vi "_053.vi"() -> ()   [LabVIEW 2024]
uses:
  <vilib>/Math Plots/3D Math Plots/3D Bar/3D Bar XCtrl/3D Bar.xctl
  <vilib>/Math Plots/3D Math Plots/3D Bar/3D Bar Datatype/Public/Plot Helper (Matrix).vi
  <vilib>/Math Plots/3D Math Plots/3D Bar/3D Bar Datatype/3D Bar Datatype.lvclass
panel:
  out "3D Bar":refnum<class "3D Plot Datatype.lvclass">[](xcontrol)
  # "Data plot on 3D Bar Graph :"
  # "( Sin & Cos wave , & Sinc Signal )"
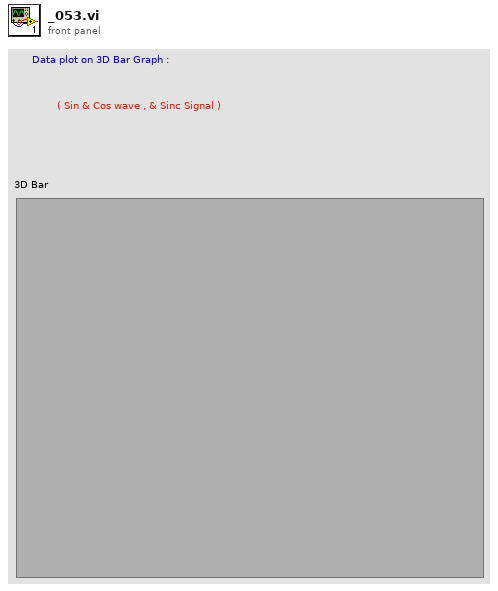
[diagram p1: front panel]
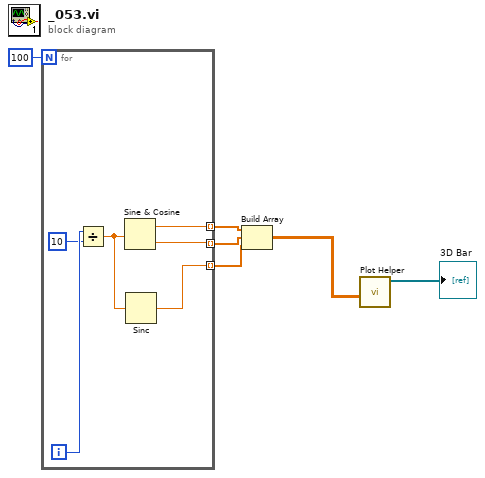
[diagram p0: block diagram]
diagram:
  n1 = for {
    N: 100 -> [_]
    tunnel: [w12] -> w4 mode=indexing
    tunnel: [w11] -> w3 mode=indexing
    tunnel: [w7] -> w1 mode=indexing
    i -> [w10]
    n2 = Divide(x=w10, y=10) -> (x/y=w8:dbl)
    n3 = Sine & Cosine(0:w8) -> (1:w12:dbl, 2:w11:dbl)
    n4 = Sinc(1:w8) -> (0:w7:dbl)
  }
  n5 = Build Array(w4, w3, w1) -> (w2:dbl[][])
  n6 = call-poly <vilib>:"Plot Helper.vi"("z matrix"=w2) -> ("3D Plot lvclass Array out"=→"3D Bar":refnum<class "3D Plot Datatype.lvclass">[])  [unwired: 2 in, 8 out]
